vi "Setup file.vi"(8 "error in (no error)":errorcluster, 10 "Sampling data":T3 {"Channels"."Hi cutoff" items=["500"=500.0, "1k"=1000.0, "5k"=5000.0, "10k"=10000.0, "20k"=20000.0]; "Channels"."Lo cutoff" items=["0.1"=0.1, "1"=1.0, "10"=10.0, "100"=100.0, "300"=300.0]; "Channels"."Gain" items=["x100"=100, "x1000"=1000, "x10000"=10000]}, 11 "selected path":path) -> (0 "error out":errorcluster, 2 "Sampling data out":T3 {"Channels"."Hi cutoff" items=["500"=500.0, "1k"=1000.0, "5k"=5000.0, "10k"=10000.0, "20k"=20000.0]; "Channels"."Lo cutoff" items=["0.1"=0.1, "1"=1.0, "10"=10.0, "100"=100.0, "300"=300.0]; "Channels"."Gain" items=["x100"=100, "x1000"=1000, "x10000"=10000]}, 3 "file refs":T1 {"file" format="%.0x"}, 4 "path out":path)   [LabVIEW 2012]
uses:
  Sampling info.ctl
  Channel.ctl
  File refs.ctl
  <vilib>/addons/h5labview2/base/hid_t.ctl
  <vilib>/addons/h5labview2/file/H5Fmode.ctl
  <vilib>/addons/h5labview2/file/H5F.lvlib
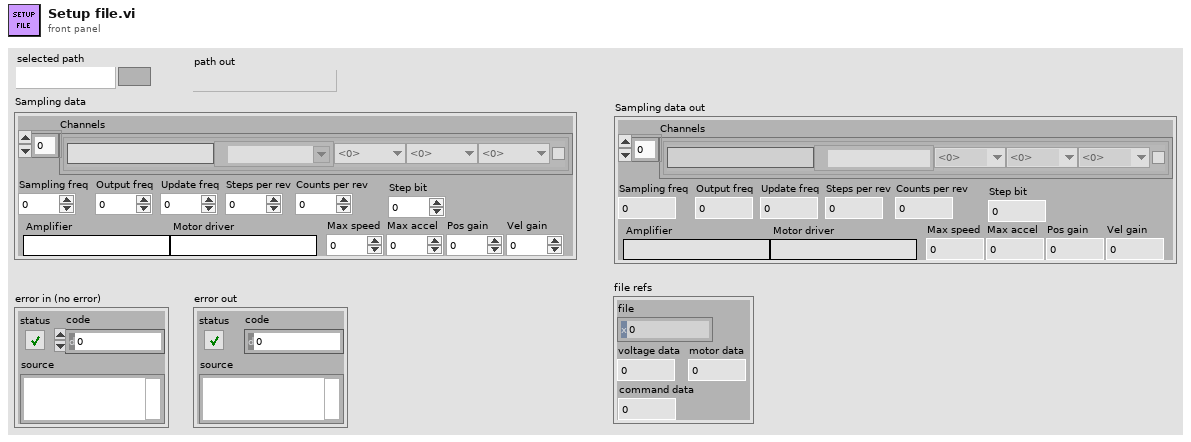
[diagram p1: front panel]
types:
  T1 = typedef "File refs.ctl" = cluster{"file":T2, "voltage data":i32, "motor data":i32, "command data":i32}
  T2 = typedef "hid_t.ctl" = i32
  T3 = typedef "Sampling info.ctl" = cluster{"Channels":T4[], "Sampling freq":i32, "Output freq":i32, "Update freq":i32, "Steps per rev":i32, "Counts per rev":i32, "Amplifier":string, "Motor driver":string, "Step bit":u8, "Max speed":dbl, "Max accel":dbl, "Pos gain":dbl, "Vel gain":dbl}
  T4 = typedef "Channel.ctl" = cluster{"Name":string, "Chan":tag, "Gain":u16, "Lo cutoff":dbl, "Hi cutoff":dbl, "Notch":bool}
  T5 = typedef "H5F.lvlib/H5Fmode.ctl" = enum16{"read-only", "read-write", "overwrite", "create new", "open or create"}
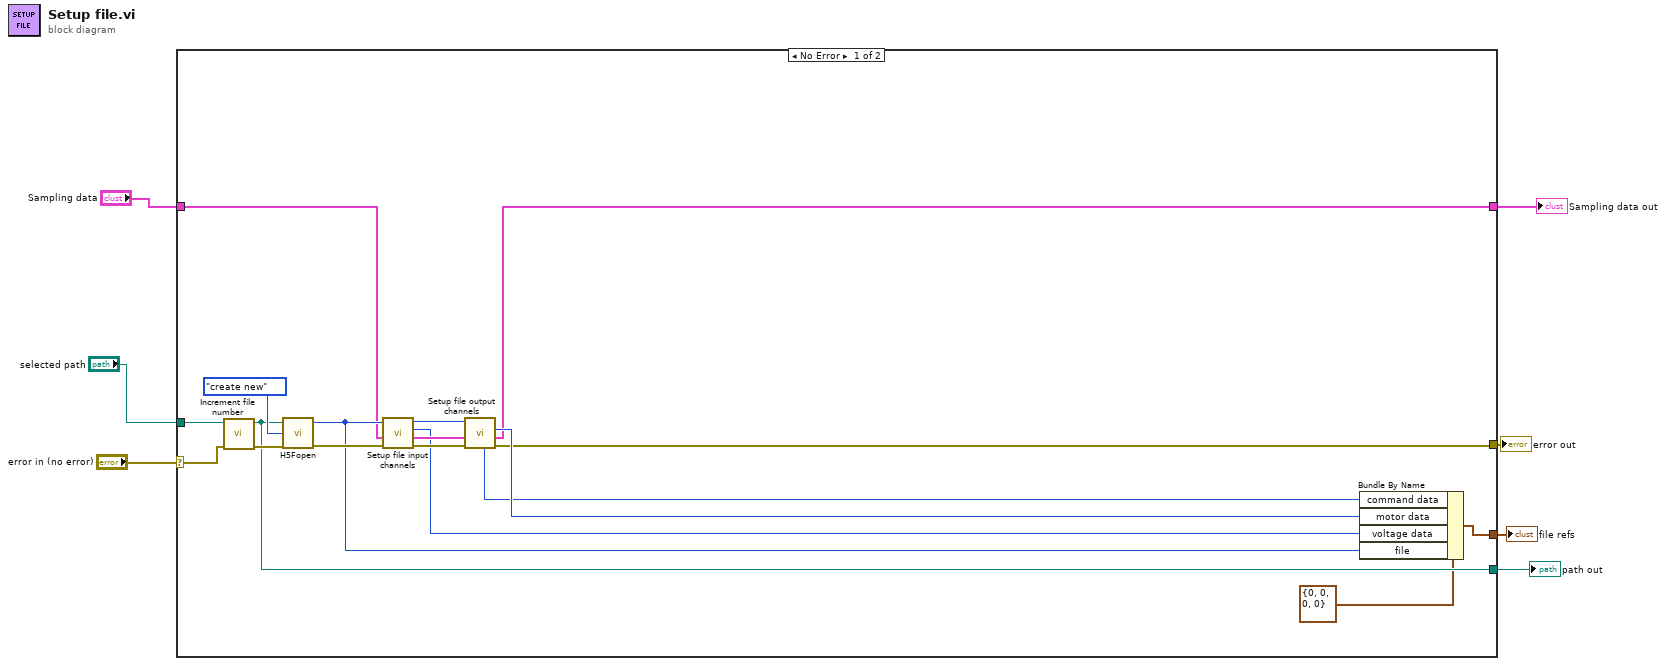
[diagram p0: block diagram]
diagram:
  n1 = case shown="No Error" "error in (no error)" {
    selector: "error in (no error)" -> [w24 w27]
    tunnel: "selected path" -> [w25 _]
    tunnel: "Sampling data" -> [w10 w26]
    tunnel: [w11 w27] -> w4
    tunnel: [w9 w26] -> w3
    tunnel: [w21 _] -> w1
    tunnel: [w20 _] -> w2
    frame No Error {
      n2 = call "Increment file number.vi"("error in"=w24, "path"=w25) -> ("error out"=w23:errorcluster, "path out"=w20:path)  [unwired: 8 in]
      n3 = call <vilib>:"H5Fopen.vi"("error in (no error)"=w23, "mode (read-only)"=H5Fmode."create new", "path"=w20) -> ("error out"=w18:errorcluster, "ref out"=w14:T2)  [unwired: 1 in]
      n4 = call "Setup file input channels.vi"("error in"=w18, "Sampling data"=w10, "file ref in"=w14) -> ("error out"=w16:errorcluster, "Sampling data out"=w15:T3, "dset ref"=w13:i32, "file ref out"=w17:T2)  [unwired: 5 in]
      n5 = call "Setup file output channels.vi"("error in"=w16, "Sampling data"=w15, "file ref in"=w17) -> ("error out"=w11:errorcluster, "Sampling data out"=w9:T3, "dset ref"=w12:i32, "cmd dset out"=w8:i32)  [unwired: 4 in, 1 out]
      n6 = Bundle By Name(cluster=T1 {"file"=0, "voltage data"=0, "motor data"=0, "command data"=0} ("file refs 2"), "command data"=w8, "motor data"=w12, "voltage data"=w13, "file"=w14) -> (w21:T1)
    }
    frame Error {
    }
  }
  "error out" <- w4
  "Sampling data out" <- w3
  "file refs" <- w1
  "path out" <- w2
